vi "Test.vi"() -> ()   [LabVIEW 2017, in "LabSFTP.lvlib"]
doc: "<License>This software is distributed under the BSD 3-Clause License. For the full license please see license.txt or visit www.labvolution.com/license</License>"
uses:
  LabSFTP.lvlib
  Connection Info..cluster.ctl
  Password..cluster.ctl
  connect_password.vi
panel:
  in  "Password":T1
  in  "Remote File Path Up":string="/home/greg/Documents/"
  in  "Local File Up":path=path "C:/Working Folder/ssh.git/Test.txt"
  in  "error in (no error)":errorcluster
  out "isSftpConnected":bool
  in  "Connection Info.":T2={"Remote"="", "Username"="", "Port (22)"=22}
  # "Upload File"
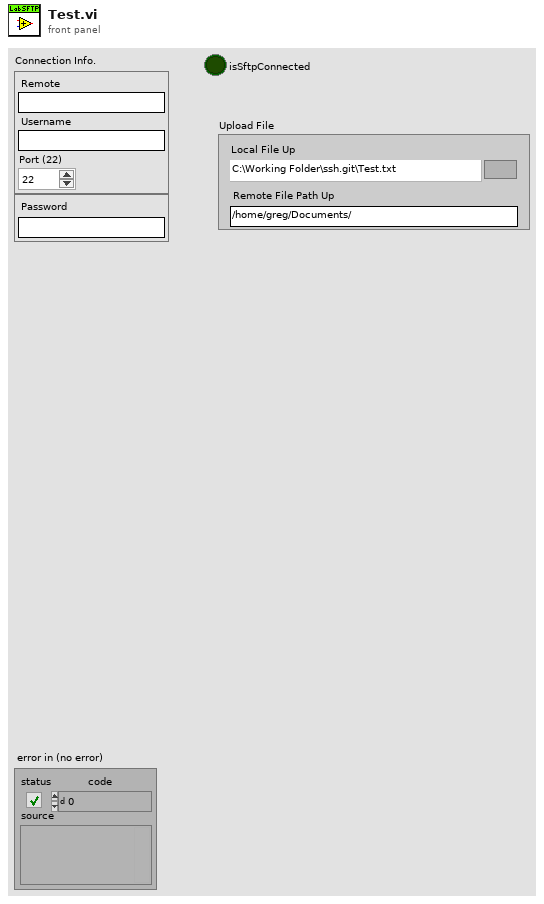
[diagram p1: front panel]
types:
  T1 = typedef "LabSFTP.lvlib/Password..cluster.ctl" = cluster{"Password":string}
  T2 = typedef "LabSFTP.lvlib/Connection Info..cluster.ctl" = cluster{"Remote":string, "Username":string, "Port (22)":i32}
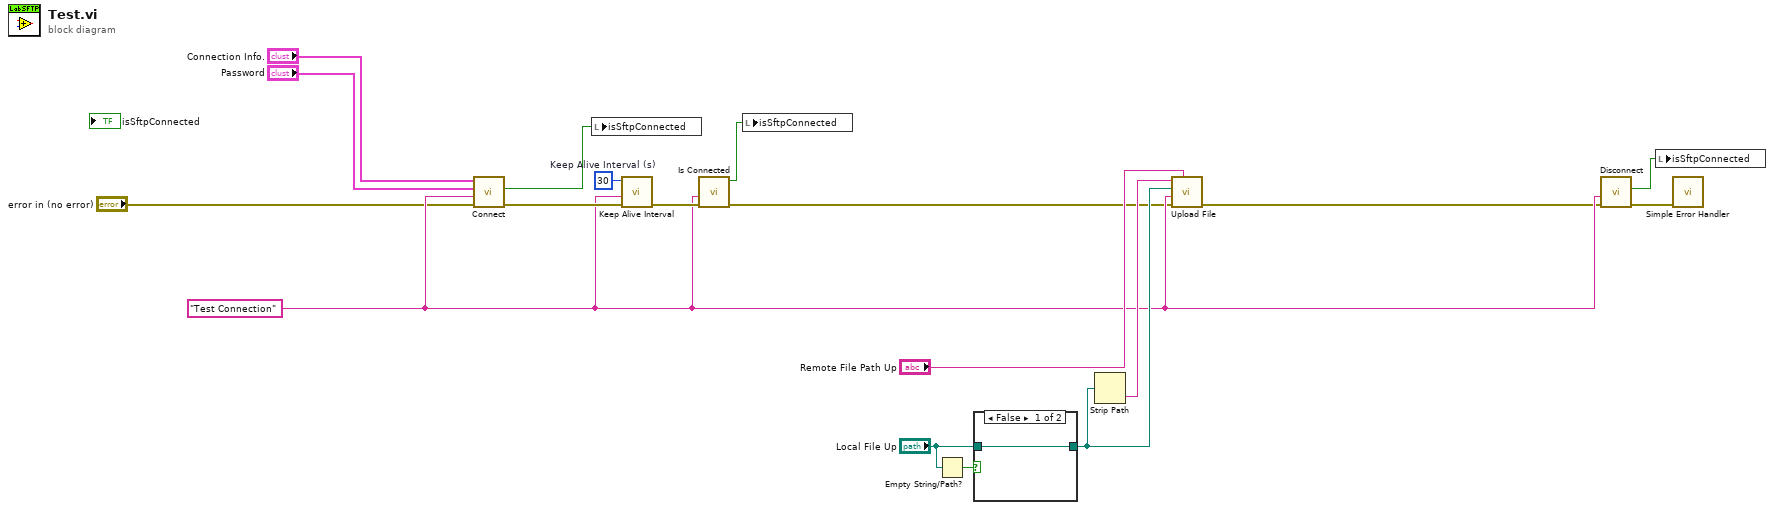
[diagram p0: block diagram]
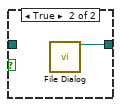
[diagram p2: hidden frame]
diagram:
  w4 = "Test Connection" ("Connection Name")
  w10 = 30  # Keep Alive Interval (s)
  n1 = call-poly "Connect.vi"("error in (no error)"="error in (no error)", "Connection Name"=w4, "Password"="Password", "Connection Info."="Connection Info.") -> ("error out"=w11:errorcluster, "isSftpConnected"=w17:bool)  [unwired: 5 in, 1 out]
  n2 = local write "isSftpConnected"(w17) -> ()
  n3 = call "Keep Alive Interval.vi"("error in (no error)"=w11, "Connection Name"=w4, "Keep Alive Interval (s)"=w10) -> ("error out"=w12:errorcluster)  [unwired: 8 in]
  n4 = call "Is Connected.vi"("error in (no error)"=w12, "Connection Name"=w4) -> ("error out"=w2:errorcluster, "isSshConnected"=w16:bool)  [unwired: 8 in]
  n5 = local write "isSftpConnected"(w16) -> ()
  n6 = Empty String/Path?(string/path="Local File Up") -> (empty?=w9:bool)
  n7 = case shown="False" w9 {
    tunnel: [w19 w20] -> w6
    tunnel: "Local File Up" -> [w19 _]
    frame False {
    }
    frame True {
      n8 = call "File Dialog"() -> ("selected path"=w20:path)  [unwired: 12 in, 3 out]
    }
  }
  n9 = Strip Path(path=w6) -> (name=w13:string)  [unwired: 1 out]
  n10 = call "Upload File.vi"("Remote Folder Path"="Remote File Path Up", "error in (no error)"=w2, "Connection Name"=w4, "Local File Path"=w6, "Remote File Name"=w13) -> ("error out"=w3:errorcluster)  [unwired: 5 in, 1 out]
  n11 = call "Disconnect.vi"("error in (no error)"=w3, "Connection Name"=w4) -> ("error out"=w15:errorcluster, "isSshConnected"=w14:bool)  [unwired: 7 in, 1 out]
  n12 = local write "isSftpConnected"(w14) -> ()
  n13 = call <vilib>:"Simple Error Handler.vi"("error in (no error)"=w15) -> ()  [unwired: 4 in, 5 out]
